vi "SR430.init.vi"(0 "i ref in":refnum<vi>, 5 "error in (no error)":errorcluster) -> (14 "i ref out":refnum<vi>, 19 "error out":errorcluster)   [LabVIEW 2014, in "SR430.lvlib"]
doc: "Initializes the SR430"
uses:
  SR430.lvlib
  CS_Core/CSSystem/CoreDefs/CoreDefs.error_type.ctl
  instr.lib/SR430/SR430Driver.lvlib
  CS_Core/CSSystem/CoreLib/CoreLib.lvlib
  CS_Core/CSApplicationBaseClasses/MCSBase/MCSBase.lvlib
  CSlibraries/UtilityLib/UtilityLib.lvlib
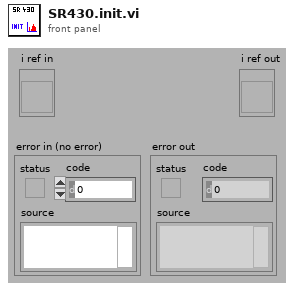
[diagram p1: front panel]
types:
  T1 = typedef "CoreDefs.error_type.ctl" = enum16{"no error", "can't load process", "can't unload process", "process does not exist", "can't install process", "can't remove process", "unknown function", "time out", "can't execute function", "duplicate queue name", "super not found", "caller queue invalid", "can't ping process", "unknown error", "VISA Error", "VISA timeout", "GPIB timeout", "GPIB error", "communication error", "data type mismatch", "can't read data from OPC server", "can't write data to OPC server", "OET error", "function not implemented", "process already exists", "invalid Shared Variable name", "error writing Shared Variable", "error reading Shared Variable", "invalid client name", "corrupt database", "unknown class", "call not authorized", "parameter out of range", "OET timeout: can't get data to modify", "invalid queue name", "requested operation incompatible with current state", "event undefined", "event disabled", "state undefined", "caller is not a friend", "EventBuilder: bad eventID", "EventBuilder: no DAQ devices", "a thread must not stop itself", "UNUSED ELEMENT4", "DiscArchiver: eventData incomplete", "DiscArchiver: eventData does not belong to run", "DiscArchiver: can't open file", "DiscArchiver: can't write to file", "DiscArchiver: available disc space low", "can't acquire semaphore", "error reading data from database", "notifier object is not existing", "can't register process", "can't unregister process", "illegal event type", "object disabled", "object already exists", "can't change state", "Instrument not found", "no connection to remote node", "invalid reference", "N/A", "UNUSED ELEMENT 1", "element not found", "illegal TCP/IP connection detected", "object does not exist", "invalid access ID", "unknown CS system", "invalid privilige", "unsupported data type", "unsupported server type", "IO server already exists", "Shared Variable already exists"}
  T2 = typedef "SR430Driver.lvlib/SR430_VISA Control.ctl" = cluster{"VISA resource name":refnum<visa-resource-name>}
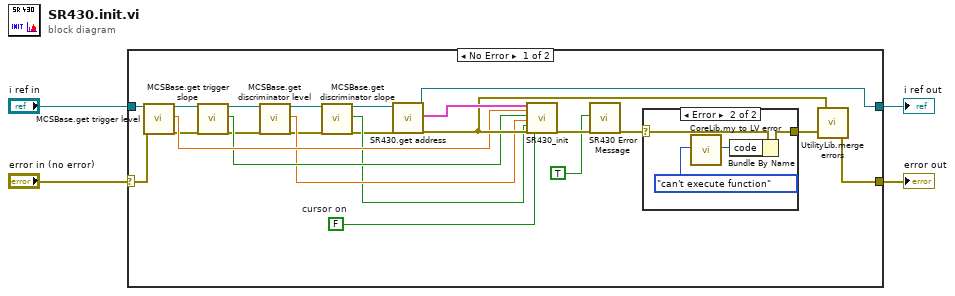
[diagram p0: block diagram]
diagram:
  n1 = case shown="No Error" "error in (no error)" {
    selector: "error in (no error)" -> [w5 w33]
    tunnel: [w24 w33] -> w4
    tunnel: [w23 w34] -> w3
    tunnel: "i ref in" -> [w22 w34]
    frame No Error {
      w25 = FALSE  # cursor on
      n2 = call "MCSBase.get trigger level.vi"("i ref in"=w22, "error in (no error)"=w5) -> ("i ref out"=w20:refnum<vi>, "triggerLevel [V]"=w21:dbl, "error out"=w19:errorcluster)  [unwired: 15 in]
      n3 = call "MCSBase.get trigger slope.vi"("i ref in"=w20, "error in (no error)"=w19) -> ("i ref out"=w17:refnum<vi>, "triggerSlope"=w18:bool, "error out"=w16:errorcluster)  [unwired: 15 in]
      n4 = call "MCSBase.get discriminator level.vi"("i ref in"=w17, "error in (no error)"=w16) -> ("i ref out"=w14:refnum<vi>, "discLevel [V]"=w15:dbl, "error out"=w13:errorcluster)  [unwired: 15 in]
      n5 = call "MCSBase.get discriminator slope.vi"("i ref in"=w14, "error in (no error)"=w13) -> ("i ref out"=w10:refnum<vi>, "discSlope"=w12:bool, "error out"=w11:errorcluster)  [unwired: 15 in]
      n6 = call "SR430.get address.vi"("i ref in"=w10, "error in (no error)"=w11) -> ("i ref out"=w23:refnum<vi>, "address"=w27:T2, "error out"=w26:errorcluster)  [unwired: 15 in]
      n7 = call "SR430_init.vi"("GPIB address"=w27, "triggeLevel [V]"=w21, "triggerSlope"=w18, "discriminatorLevel [V]"=w15, "discriminatorSlope"=w12, "error in (no error)"=w26, "cursorOn"=w25) -> ("error out"=w9:errorcluster)  [unwired: 11 in, 1 out]
      n8 = call "SR430 Error Message.vi"("addMessageToSource"=TRUE ("add message to source"), "error in (no error)"=w9) -> ("error out"=w8:errorcluster)  [unwired: 14 in, 3 out]
      n9 = case shown="Error" w8 {
        selector: w8 -> [w28 w32]
        tunnel: [w28 w29] -> w6
        frame No Error {
        }
        frame Error {
          n10 = call "CoreLib.my to LV error.vi"("ErrorTypes"=CoreDefs.error_type."can't execute function") -> ("LV error code"=w31:i32)  [unwired: 17 in, 1 out]
          n11 = Bundle By Name(cluster=w32, "code"=w31) -> (w29:errorcluster)
        }
      }
      n12 = call "UtilityLib.merge errors.vi"("error2 (no error)"=w6, "error1 (no error)"=w26) -> ("error out"=w24:errorcluster)
    }
    frame Error {
    }
  }
  "error out" <- w4
  "i ref out" <- w3
